vi "PostCopyScripting.vi"(10 "MetaDataObj":refnum<class "MetaDataObj.lvclass">, 11 "User Project":refnum<vi>) -> ()   [LabVIEW 2013, in "editorscriptingobjectBasicExec.lvclass"]
uses:
  editorscriptingobjectBasicExec.lvclass
  <resource>/dialog/NewProjectWizard/MetaDataObj/MetaDataObj.lvclass
  <vilib>/Utility/EditLVLibs/Edit LVLibs.lvlib
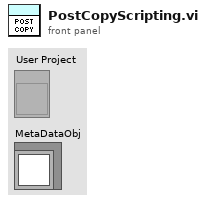
[diagram p1: front panel]
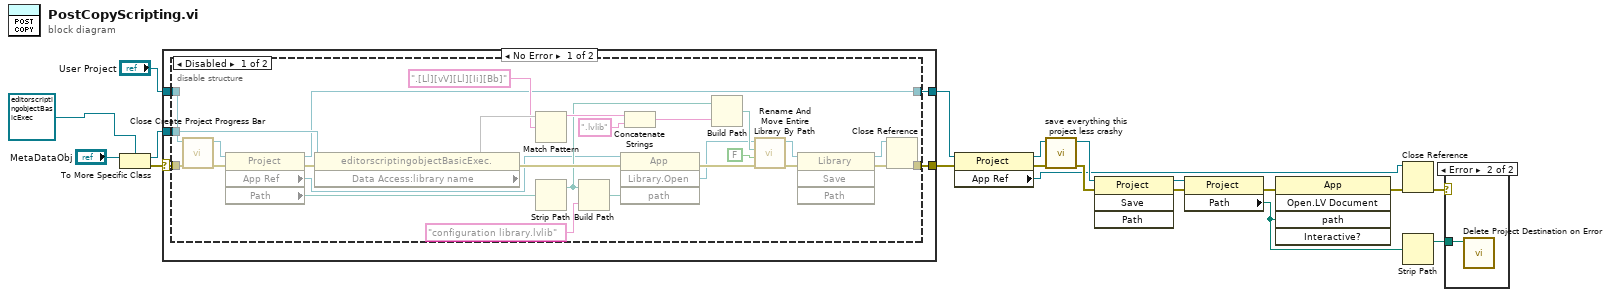
[diagram p0: block diagram]
diagram:
  n1 = To More Specific Class(target class=refnum<class "editorscriptingobjectBasicExec.lvclass"> refnum ("editorscriptingobjectBasicExec.lvclass"), reference="MetaDataObj") -> (specific class reference=w11:refnum<class "editorscriptingobjectBasicExec.lvclass">, error out=w18:errorcluster)  [unwired: 1 in]
  n2 = case shown="No Error" w18 {
    selector: w18 -> [w23 w54]
    tunnel: [w20 w55] -> w8
    tunnel: "User Project" -> [w22 w55]
    tunnel: [w21 w54] -> w7
    tunnel: w11 -> [w24 _]
    frame No Error {
      n3 = disable-structure shown="Disabled" {
        disable-tunnel: w24 -> [w49 _]
        disable-tunnel: w23 -> [w48 w52]
        disable-tunnel: w22 -> [w47 w53]
        disable-tunnel: [w26 w52] -> w21
        disable-tunnel: [w25 w53] -> w20
        frame Disabled {
          n4 = call <resource>:"Close Create Project Progress Bar.vi"("error in (no error)"=w48, "Project"=w47) -> ("error out"=w45:errorcluster, "dup Project"=w46:refnum<vi>)  [unwired: 8 in]
          n5 = property class="Project"(reference=w46, error in=w45) -> (reference out=w25:refnum<vi>, error out=w51:errorcluster, "App Ref"=w35:refnum<vi>, "Path"=w50:path)
          n6 = property class="editorscriptingobjectBasicExec."(reference=w49, error in=w51) -> (error out=w43:errorcluster, "Data Access:library name"=w42)  [unwired: 1 out]
          n7 = Match Pattern(string=w42, regular expression=".[Ll][vV][Ll][Ii][Bb]") -> (before substring=w40:string)  [unwired: 1 in, 3 out]
          n8 = Strip Path(path=w50) -> (stripped path=w37:path)  [unwired: 1 out]
          n9 = Build Path(base path=w37, name or relative path="configuration library.lvlib") -> (appended path=w34:path)
          n10 = invoke class="App" method="Library.Open"(reference=w35, error in=w43, "path"=w34) -> (error out=w36:errorcluster, "Open Library"=w32:refnum<vi>)  [unwired: 1 in, 2 out]
          n11 = Concatenate Strings(w40, ".lvlib" ("string")) -> (w38:string)
          n12 = Build Path(base path=w37, name or relative path=w38) -> (appended path=w33:path)
          n13 = call <vilib>:"Rename And Move Entire Library By Path.vi"("error in (no error)"=w36, "Delete old directory if empty after move? (T)"=FALSE, "New library path"=w33, "Library ref in"=w32) -> ("error out"=w30:errorcluster, "Library ref out"=w29:refnum<vi>)  [unwired: 6 in]
          n14 = invoke class="Library" method="Save"(reference=w29, error in=w30) -> (reference out=w27:refnum<vi>, error out=w28:errorcluster)  [unwired: 2 in, 2 out]
          n15 = Close Reference(reference=w27, error in (no error)=w28) -> (error out=w26:errorcluster)
        }
        frame Enabled {
        }
      }
    }
    frame Error {
    }
  }
  n16 = property class="Project"(reference=w8, error in=w7) -> (reference out=w5:refnum<vi>, error out=w6:errorcluster, "App Ref"=w4:refnum<vi>)
  n17 = call "save everything this project less crashy.vi"("error in"=w6, "Project in"=w5) -> ("error out"=w10:errorcluster, "Project out"=w9:refnum<vi>)  [unwired: 8 in]
  n18 = invoke class="Project" method="Save"(reference=w9, error in=w10) -> (reference out=w14:refnum<vi>, error out=w15:errorcluster)  [unwired: 2 in, 2 out]
  n19 = property class="Project"(reference=w14, error in=w15) -> (error out=w17:errorcluster, "Path"=w12:path)  [unwired: 1 out]
  n20 = invoke class="App" method="Open.LV Document"(error in=w17, "path"=w12) -> (error out=w16:errorcluster)  [unwired: 3 in, 4 out]
  n21 = Close Reference(reference=w4, error in (no error)=w16) -> (error out=w3:errorcluster)
  n22 = Strip Path(path=w12) -> (stripped path=w2:path)  [unwired: 1 out]
  n23 = case shown="Error" w3 {
    tunnel: w2 -> [_ w56]
    frame No Error {
    }
    frame Error {
      n24 = call <resource>:"Delete Project Destination on Error.vi"("Project Destination Root"=w56) -> ()  [unwired: 11 in]
    }
  }
